vi "CCP_tcp_client.vi"(6 "close_tcp":bool=TRUE, 7 "wait_time":i32=1000, 8 "error in":errorcluster, 9 "port":u16=9999, 10 "address":string="127.0.0.1", 11 "conn_id_in":refnum<k5>) -> (0 "error out":errorcluster, 1 "array_value":dbl[](array[numeric]), 2 "status":bool, 3 "conn_id_out":refnum<k5>)   [LabVIEW 2019]
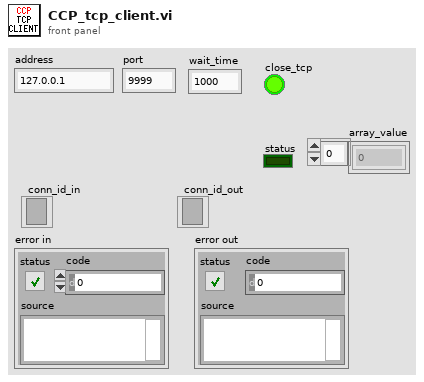
[diagram p1: front panel]
types:
  T1 = enum16{"Standard", "Buffered", "CRLF", "Immediate"}
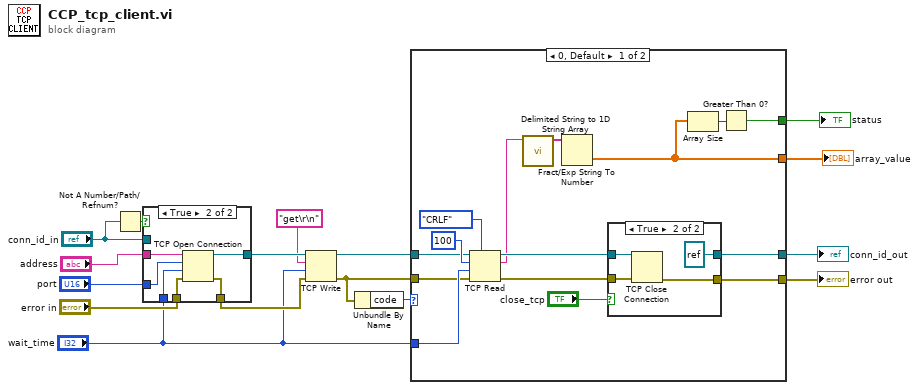
[diagram p0: block diagram]
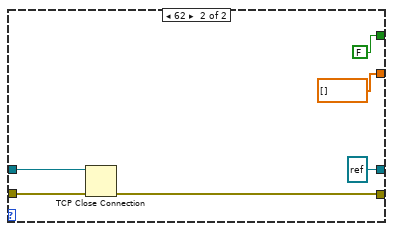
[diagram p3: hidden frame]
diagram:
  n1 = Not A Number/Path/Refnum?(number/path/refnum="conn_id_in") -> (NaN/Path/Refnum?=w15:bool)
  n2 = case shown="True" w15 {
    tunnel: "port" -> [_ w20]
    tunnel: "address" -> [_ w24]
    tunnel: [w17 w23] -> w8
    tunnel: [w18 w22] -> w10
    tunnel: "conn_id_in" -> [w18 _]
    tunnel: "error in" -> [w17 w21]
    tunnel: "wait_time" -> [_ w19]
    frame False {
    }
    frame True {
      n3 = TCP Open Connection(address=w24, remote port or service name=w20, timeout ms (60000)=w19, error in (no error)=w21) -> (connection ID=w22:refnum<k5>, error out=w23:errorcluster)  [unwired: 1 in]
    }
  }
  n4 = TCP Write(connection ID=w10, data in="get\r\n", error in (no error)=w8, 9:"wait_time") -> (connection ID out=w6:refnum<k5>, error out=w3:errorcluster)  [unwired: 1 out]
  n5 = Unbundle By Name(w3) -> ("code"=w2:i32)
  n6 = case shown="0, Default" w2 {
    tunnel: [w28 FALSE] -> w16
    tunnel: "wait_time" -> [w35 _]
    tunnel: w6 -> [w34 w47]
    tunnel: [w32 refnum<k5> refnum ("connection ID")] -> w5
    tunnel: [w31 w46] -> w4
    tunnel: w3 -> [w30 w48]
    tunnel: [w25 dbl[] []] -> w1
    frame 0, Default {
      n7 = TCP Read(connection ID=w34, bytes to read=100, error in (no error)=w30, 7:T1."CRLF" ("mode (standard)"), 9:w35) -> (connection ID out=w38:refnum<k5>, data out=w27:string, error out=w39:errorcluster)
      n8 = call <vilib>:"Delimited String to 1D String Array.vi"("delimited string"=w27) -> ("string array"=w26:string[])  [unwired: 10 in]
      n9 = Fract/Exp String To Number(string=w26) -> (number=w25:dbl[])  [unwired: 3 in, 1 out]
      n10 = case shown="True" "close_tcp" {
        tunnel: w39 -> [w40 w45]
        tunnel: w38 -> [w41 w44]
        tunnel: [w40 w43] -> w31
        tunnel: [w41 refnum<k5> refnum ("connection ID")] -> w32
        frame False {
        }
        frame True {
          n11 = TCP Close Connection(connection ID=w44, error in (no error)=w45) -> (error out=w43:errorcluster)  [unwired: 1 in, 1 out]
        }
      }
      n12 = Array Size(array=w25) -> (size(s)=w29:i32)
      n13 = Greater Than 0?(x=w29) -> (x > 0?=w28:bool)
    }
    frame 62 {
      n14 = TCP Close Connection(connection ID=w47, error in (no error)=w48) -> (error out=w46:errorcluster)  [unwired: 1 in, 1 out]
    }
  }
  "status" <- w16
  "conn_id_out" <- w5
  "error out" <- w4
  "array_value" <- w1
